vi "List Buckets.vi"(8 "error in (no error)":errorcluster, 11 "AWS Credentials":T1) -> (0 "error out":errorcluster, 1 "Owner display name":string, 2 "Owner ID":string, 3 "Buckets":refnum<class "Bucket.lvclass">[](array[class]))   [LabVIEW 2015, in "NI_AWS_S3.lvlib" / "Bucket.lvclass"]
doc: "List the buckets for the specified account. This requires the ListAllMyBuckets permission for the account."
uses:
  Bucket.lvclass
  Core/HTTP Request/AWS Credentials.ctl
  Core/HTTP Request/Request Options.ctl
  Core/HTTP Request/Name Value Pair.ctl
  Core/HTTP Request/Region handling.ctl
  Core/HTTP Request/URL formatting.ctl
  Core/HTTP Request/HTTP Request.lvclass/HTTP Request.ctl
  Bucket.lvclass/Bucket.ctl
  Write Name.vi
  Write Creation Date.vi
  Core/HTTP Request/Write Verify Server.vi
  Core/HTTP Request/Write Credentials.vi
  Core/HTTP Request/Write Service.vi
  Core/HTTP Request/HTTP Request.lvclass
  XML Parsing/NI_XML Parsing.lvlib
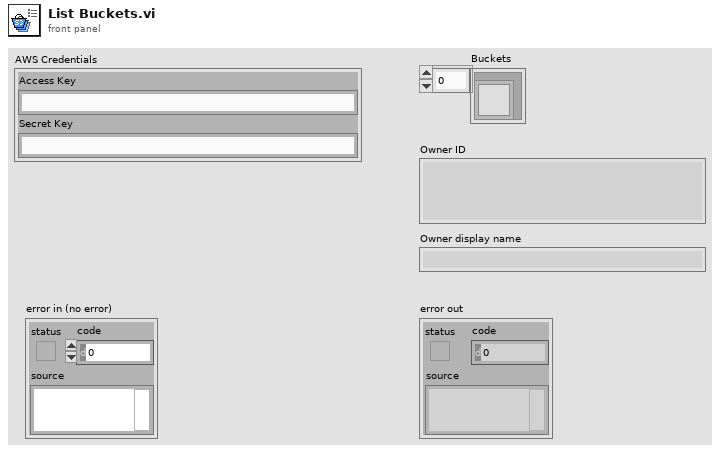
[diagram p1: front panel]
types:
  T1 = typedef "NI_AWS_Core.lvlib/HTTP Request.lvclass/AWS Credentials.ctl" = cluster{"Access Key":string, "Secret Key":string}
  T2 = typedef "NI_AWS_Core.lvlib/HTTP Request.lvclass/Region handling.ctl" = enum16{"use region everywhere", "use region (authentication only)", "use region (URL only)", "ignore region everwhere"}
  T3 = typedef "NI_AWS_Core.lvlib/HTTP Request.lvclass/Request Options.ctl" = cluster{"request headers":T4[], "request parameters":T4[], "request body":string, "region handling":T2, "URL formatting":T5}
  T4 = typedef "NI_AWS_Core.lvlib/HTTP Request.lvclass/Name Value Pair.ctl" = cluster{"name":string, "value":string}
  T5 = typedef "NI_AWS_Core.lvlib/HTTP Request.lvclass/URL formatting.ctl" = enum16{"region-", "region."}
  T6 = typedef "NI_AWS_Core.lvlib/HTTP Request.lvclass/Response.ctl" = cluster{"Headers":string, "Body":string}
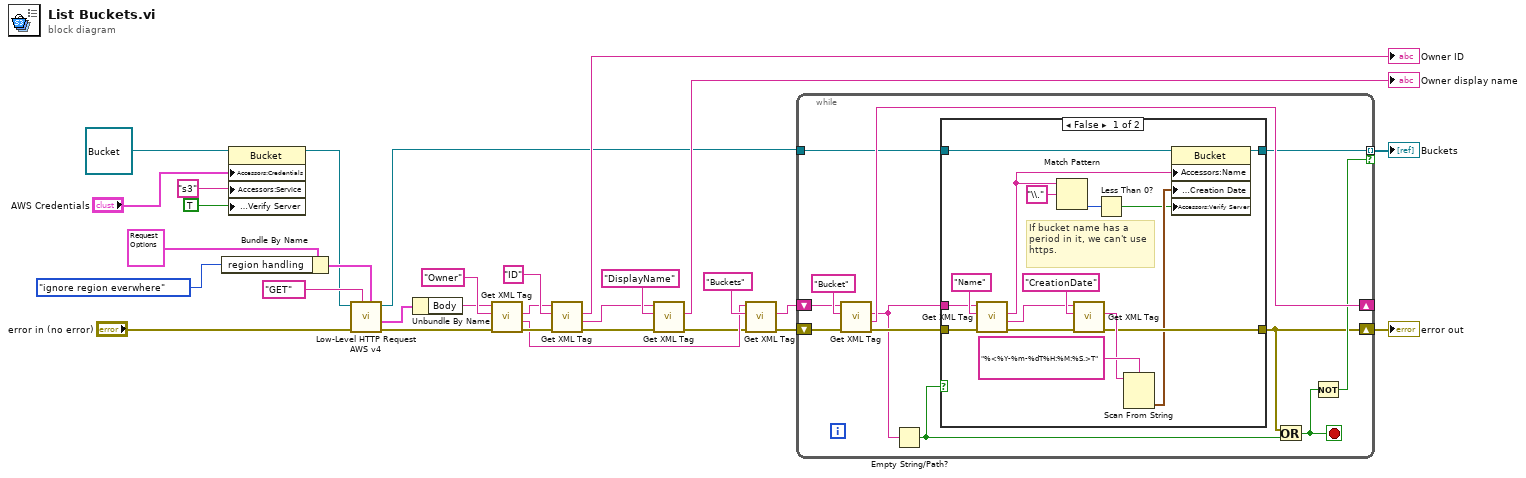
[diagram p0: block diagram]
diagram:
  n1 = Bundle By Name(cluster=T3 {"request headers"=[], "request parameters"=[], "request body"="", "region handling"=enum."use region everywhere", "URL formatting"=enum."region."} ("Request Options"), "region handling"=Region_handling."ignore region everwhere") -> (w4:T3)
  n2 = property class="Bucket"(reference=refnum<class "Bucket.lvclass"> refnum ("NI_AWS_S3.lvlib:Bucket.lvclass"), "Accessors:Credentials"="AWS Credentials", "Accessors:Service"="s3" ("Service"), "Accessors:Verify Server"=TRUE ("Verify Server")) -> (reference out=w1:refnum<class "Bucket.lvclass">)  [unwired: 1 in, 1 out]
  n3 = call "Low-Level HTTP Request AWS v4.vi"("Request Options"=w4, "HTTP-Verb"="GET", "error in (no error)"="error in (no error)", "AWS Core in"=w1) -> ("error out"=w9:errorcluster, "Response"=w5:T6, "AWS Core out"=w2:refnum<class "Bucket.lvclass">)  [unwired: 4 in, 1 out]
  n4 = Unbundle By Name(w5) -> ("Body"=w16:string)
  n5 = call "Get XML Tag.vi"("error in (no error)"=w9, "Tag name"="Owner", "XML String in"=w16) -> ("error out"=w19:errorcluster, "Remaining string"=w15:string, "Tag value"=w17:string)  [unwired: 4 in, 2 out]
  n6 = call "Get XML Tag.vi"("error in (no error)"=w19, "Tag name"="ID", "XML String in"=w17) -> ("error out"=w18:errorcluster, "Remaining string"=w14:string, "Tag value"=→"Owner ID":string)  [unwired: 4 in, 2 out]
  n7 = call "Get XML Tag.vi"("error in (no error)"=w18, "Tag name"="DisplayName", "XML String in"=w14) -> ("error out"=w10:errorcluster, "Tag value"=→"Owner display name":string)  [unwired: 4 in, 3 out]
  n8 = call "Get XML Tag.vi"("error in (no error)"=w10, "Tag name"="Buckets", "XML String in"=w15) -> ("error out"=w24:errorcluster, "Tag value"=w13:string)  [unwired: 4 in, 3 out]
  n9 = while {
    shift-right: [w38] -> _
    shift-left: w13 -> [w41]
    shift-right: [w34] -> w20
    shift-left: w24 -> [w40]
    tunnel: w2 -> [w36]
    tunnel: [w31] -> w8 mode=indexing if=w35
    stop <- w32 stop-if-true
    n10 = call "Get XML Tag.vi"("error in (no error)"=w40, "Tag name"="Bucket", "XML String in"=w41) -> ("error out"=w39:errorcluster, "Remaining string"=w38:string, "Tag value"=w37:string)  [unwired: 4 in, 2 out]
    n11 = Empty String/Path?(string/path=w37) -> (empty?=w33:bool)
    n12 = case shown="False" w33 {
      tunnel: w39 -> [w53 w59]
      tunnel: [w49 w59] -> w34
      tunnel: w37 -> [w52 _]
      tunnel: w36 -> [w51 _]
      tunnel: [w48 _] -> w31
      frame False {
        # "If bucket name has a period in it, we can't use https."
        n13 = call "Get XML Tag.vi"("error in (no error)"=w53, "Tag name"="Name", "XML String in"=w52) -> ("error out"=w54:errorcluster, "Remaining string"=w50:string, "Tag value"=w46:string)  [unwired: 4 in, 2 out]
        n14 = Match Pattern(string=w46, regular expression="\\.") -> (offset past match=w44:i32)  [unwired: 1 in, 3 out]
        n15 = call "Get XML Tag.vi"("error in (no error)"=w54, "Tag name"="CreationDate", "XML String in"=w50) -> ("error out"=w49:errorcluster, "Tag value"=w55:string)  [unwired: 4 in, 3 out]
        n16 = Less Than 0?(x=w44) -> (x < 0?=w43:bool)
        n17 = Scan From String(format string="%<%Y-%m-%dT%H:%M:%S.>T", input string=w55) -> (output 1=w47:timestamp)  [unwired: 3 in, 3 out]
        n18 = property class="Bucket"(reference=w51, "Accessors:Name"=w46, "Accessors:Creation Date"=w47, "Accessors:Verify Server"=w43) -> (reference out=w48:refnum<class "Bucket.lvclass">)  [unwired: 1 in, 1 out]
      }
      frame True {
      }
    }
    n19 = Or(x=w34, y=w33) -> (x .or. y?=w32:bool)
    n20 = Not(x=w32) -> (.not. x?=w35:bool)
  }
  "error out" <- w20
  "Buckets" <- w8
